vi "flatten_scope_config.vi"(8 "error in (no error)":errorcluster, 10 "scope_config":T1={"VISA"="lecroy", "channels"=[enum."Channel 1"], "timeout (ms)"=100000, "max_points"=2500, "averages"=50, "noise filter"=enum."None"} {"averages" min=1; "max_points" items=["50"=50, "100"=100, "250"=250, "500"=500, "1000"=1000, "2500"=2500, "5K"=5000, "10K"=10000, "25K"=25000, "50K"=50000, "100K"=100000, "250K"=250000, "500K"=500000, "1M"=1000000, "2M"=2000000, "2.5M"=2500000, "5M"=5000000, "10M"=10000000, "25M"=25000000, "50M"=50000000, "100M"=100000000]}, 11 "name":string="scope_") -> (0 "error out":errorcluster, 1 "values":variant[](array[variant]), 2 "names":string[](array[string]))   [LabVIEW 2017, in "tools.lvlib"]
uses:
  hardware/lecroy/scope_config.ctl
  <vilib>/Utility/VariantDataType/GetClusterInfo.vi
  <vilib>/Utility/VariantDataType/GetTypeInfo.vi
  <vilib>/UPVI/lvhdf5/attribute.llb/Cluster to Attribute Array.xnode
  tools.lvlib
  <vilib>/Utility/VariantDataType/VariantType.lvlib
  hardware/lecroy/lecroy.lvlib
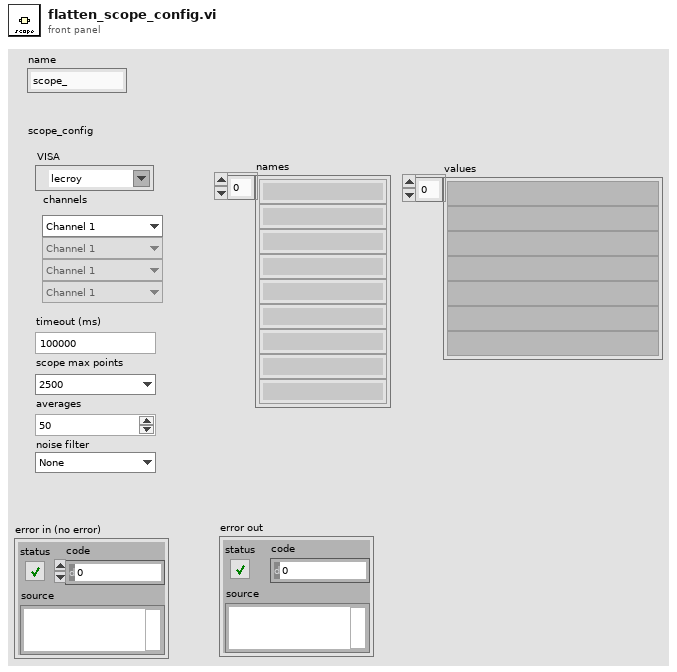
[diagram p1: front panel]
types:
  T1 = typedef "lecroy.lvlib/scope_config.ctl" = cluster{"VISA":refnum<visa-resource-name>, "channels":enum16{"Channel 1", "Channel 2", "Channel 3", "Channel 4"}[], "timeout (ms)":u32, "max_points":i32, "averages":i32, "noise filter":enum16{"None", "+0.5 bit", "+1 bit", "+1.5 bits", "+2 bits", "+2.5 bits", "+3 bits"}}
  T2 = enum16{"Channel 1", "Channel 2", "Channel 3", "Channel 4"}[]
  T3 = enum16{"None", "+0.5 bit", "+1 bit", "+1.5 bits", "+2 bits", "+2.5 bits", "+3 bits"}
  T4 = cluster{"VISA":string, "channels":enum16{"Channel 1", "Channel 2", "Channel 3", "Channel 4"}[], "timeout (ms)":u32, "max_points":i32, "averages":i32, "noise filter":enum16{"None", "+0.5 bit", "+1 bit", "+1.5 bits", "+2 bits", "+2.5 bits", "+3 bits"}}
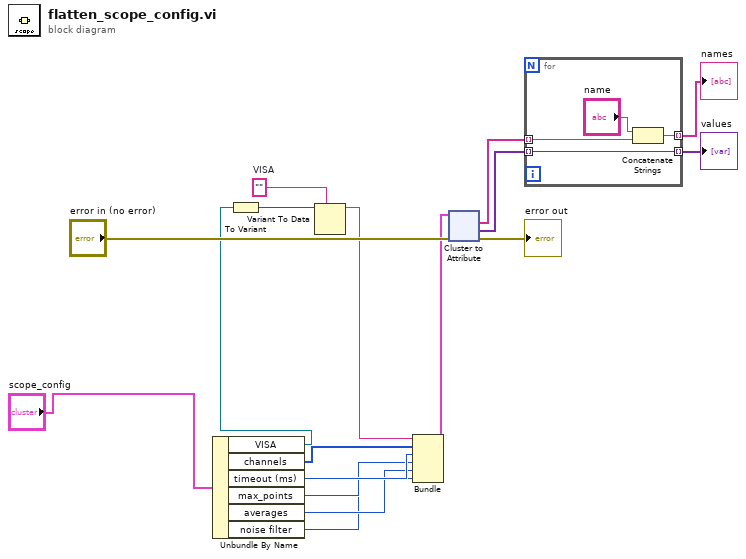
[diagram p0: block diagram]
diagram:
  w11 = ""  # VISA
  n1 = Unbundle By Name("scope_config") -> ("VISA"=w3:refnum<visa-resource-name>, "channels"=w8:T2, "timeout (ms)"=w7:u32, "max_points"=w6:i32, "averages"=w5:i32, "noise filter"=w4:T3)
  n2 = To Variant(anything=w3) -> (Variant=w10:variant)
  n3 = Variant To Data(type=w11, Variant=w10) -> (data=w2:string)  [unwired: 1 in, 1 out]
  n4 = Bundle("VISA"=w2, "channels"=w8, "timeout (ms)"=w7, "max_points"=w6, "averages"=w5, "noise filter"=w4) -> (w1:T4)  [unwired: 1 in]
  n5 = xnode "Cluster to Attribute"("error in (no error)"="error in (no error)", "Cluster"=w1) -> ("Names out"=w17:string[], "Values out"=w16:variant[], "error out"=→"error out":errorcluster)  [unwired: 4 in]
  n6 = for {
    tunnel: w17 -> [w21] mode=indexing
    tunnel: [w20] -> w15 mode=indexing
    tunnel: w16 -> [w19] mode=indexing
    tunnel: [w19] -> w14 mode=indexing
    n7 = Concatenate Strings("name", w21) -> (w20:string)
  }
  "values" <- w14
  "names" <- w15
